vi "Register.vi"(9 "subchannel":i32, 10 "element (unused)":cluster{"cmd":string, "data":variant}, 11 "data in":refnum<class "EventMessengerMData.lvclass">) -> (2 "event registration refnum":refnum<event-registration>, 3 "data out":refnum<class "EventMessengerMData.lvclass">)   [LabVIEW 2019, in "Event MessengerM.lvlib" / "EventMessengerMData.lvclass"]
uses:
  EventMessengerMData.lvclass
  EventMessengerMData.lvclass/EventMessengerMData.ctl
  <vilib>/Utility/miscctls.llb/LVMapReplaceAction.ctl
  Event Data.ctl
  Event MessengerM.lvlib
panel:
  # "See note on block diagram."
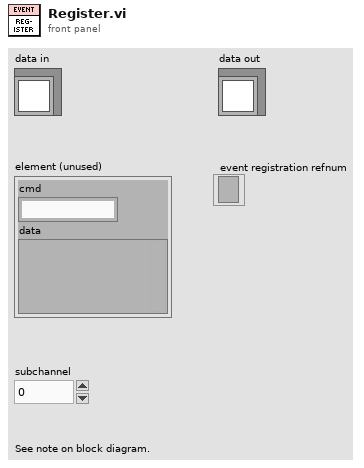
[diagram p1: front panel]
types:
  T1 = typedef "LVMapReplaceAction.ctl" = enum32{"Modify Entry only if found", "Add or Modify Entry", "Delete Entry"}
  T2 = map{i32, cluster{"Write Count":u32, "Reg Refnum":u32, "aborted?":bool, "last element?":bool, "Event Refnum":refnum<user-event>}}
  T3 = cluster{"Write Count":u32, "Reg Refnum":u32, "aborted?":bool, "last element?":bool, "Event Refnum":refnum<user-event>}
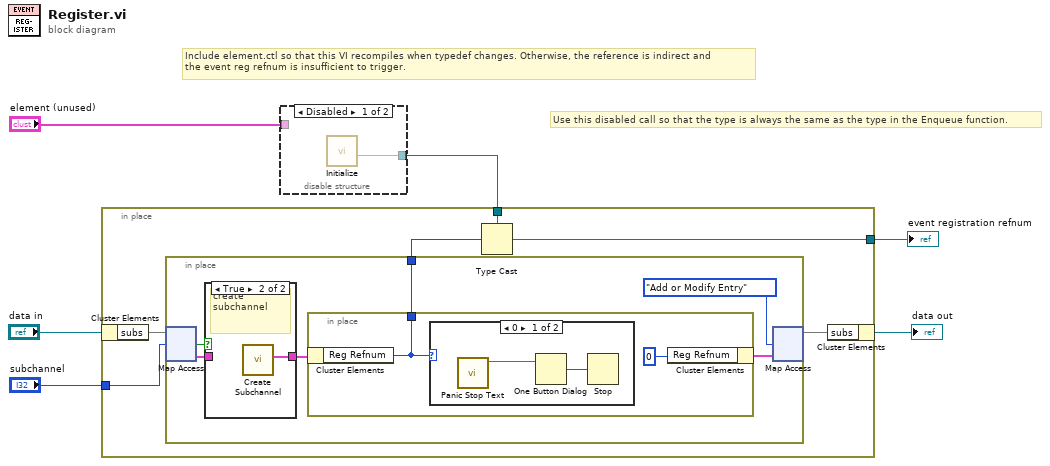
[diagram p0: block diagram]
diagram:
  # "Include element.ctl so that this VI recompiles when typedef changes. Otherwise, the reference is indirect and\nthe event reg refnum is insufficient to trigger."
  # "Use this disabled call so that the type is always the same as the type in the Enqueue function."
  n1 = disable-structure shown="Disabled" {
    disable-tunnel: [w7 _] -> w6
    disable-tunnel: "element (unused)" -> [_ _]
    frame Disabled {
      n2 = call "Initialize.vi"() -> ("Event Registration Refnum"=w7:refnum<event-registration>)  [unwired: 10 in, 1 out]
    }
    frame Enabled {
    }
  }
  n3 = in-place {
    in-place-border: w6 -> [w13]
    in-place-border: [w12] -> w1
    in-place-border: "subchannel" -> [w9]
    n4 = in-place-cluster #1("data in") -> ("subs"=w10:T2)
    n5 = in-place {
      in-place-border: [w19] -> w11
      n6 = in-place-map #2(w10, w9) -> (w16:T3, w17:bool)  [unwired: 1 in]
      n7 = case shown="True" w17 {
        tunnel: w16 -> [w20 _]
        tunnel: [w20 w21] -> w14
        frame False {
          # "subchannel exists"
        }
        frame True {
          # "create subchannel"
          n8 = call "Create Subchannel.vi"() -> ("subchannel"=w21:T3)  [unwired: 10 in, 1 out]
        }
      }
      n9 = in-place {
        in-place-border: [w22] -> w19
        n10 = in-place-cluster #3(w14) -> ("Reg Refnum"=w22:u32)
        n11 = case shown="0" w22 {
          frame 0 {
            n12 = call "Panic Stop Text.vi"() -> ("Text"=w24:string)  [unwired: 11 in]
            n13 = One Button Dialog(message=w24) -> (true=w25:bool)  [unwired: 1 in]
            n14 = Stop(stop? (T)=w25) -> ()
          }
          frame Default {
          }
        }
        n15 = in-place-cluster #3("Reg Refnum"=u32 0) -> (w18:T3)
      }
      n16 = in-place-map #2(w18, LVMapReplaceAction."Add or Modify Entry" ("action")) -> (w8:T2)  [unwired: 2 out]
    }
    n17 = Type Cast(type=w13, x=w11) -> (*(type *) &x=w12:refnum<event-registration>)
    n18 = in-place-cluster #1("subs"=w8) -> (→"data out":refnum<class "EventMessengerMData.lvclass">)
  }
  "event registration refnum" <- w1
